vi "Delete from Array.vi"   [LabVIEW 2016, in "JSON Value.lvclass"]
doc: "Deletes an element or subarray from a JSON array of length elements starting at index. Returns the edited array in array w/ subset deleted and the deleted element or subarray in deleted portion."
uses:
  JSON Helper/JSON Value.lvclass
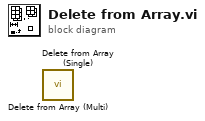
[diagram p0: block diagram]
diagram:
  n1 = call "Delete from Array (Multi).vi"() -> ()  [unwired: 10 in, 2 out]
  n2 = call "Delete from Array (Single).vi"() -> ()  [unwired: 10 in, 2 out]
